vi "Find Channel.vi"(6 "Set":bool, 8 "error in":errorcluster, 10 "Name in":string, 11 "MLTFNC in":refnum<class "MLTFNC.lvclass">) -> (0 "error out":errorcluster, 3 "MLTFNC out":refnum<class "MLTFNC.lvclass">)   [LabVIEW 2019, in "MLTFNC.lvlib" / "MLTFNC.lvclass"]
uses:
  Library/MLTFNC.lvclass
  Library/MLTFNC.lvclass/MLTFNC.ctl
  Accessors/Read Names.vi
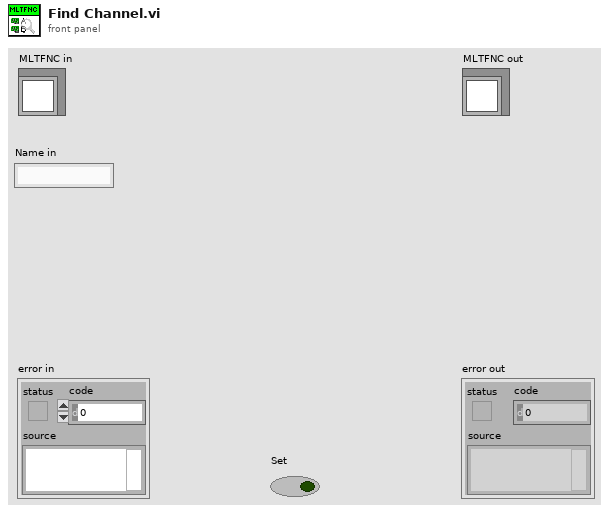
[diagram p1: front panel]
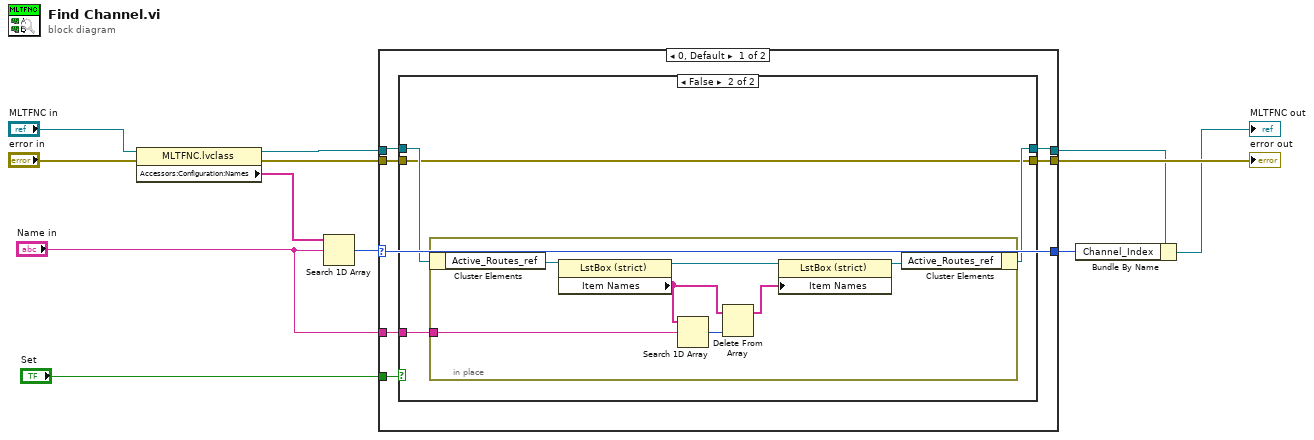
[diagram p0: block diagram]
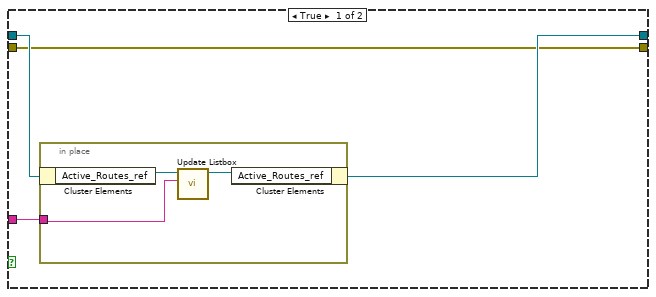
[diagram p2: hidden frame]
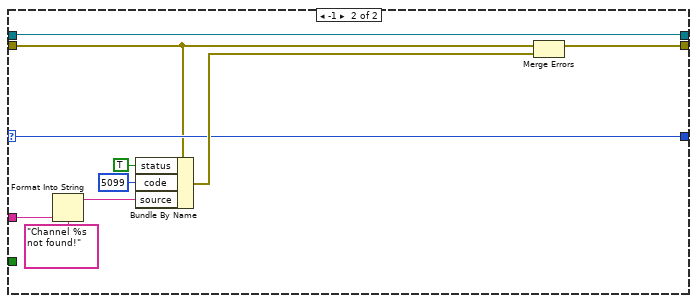
[diagram p3: hidden frame]
diagram:
  n1 = property class="MLTFNC.lvclass"(reference="MLTFNC in", error in="error in") -> (reference out=w5:refnum<class "MLTFNC.lvclass">, error out=w12:errorcluster, "Accessors:Configuration:Names"=w10:string[])
  n2 = Search 1D Array(1D array=w10, element="Name in") -> (index of element=w11:i32)  [unwired: 1 in]
  n3 = case shown="0, Default" w11 {
    selector: w11 -> [w19 w41]
    tunnel: [w19 w41] -> w2
    tunnel: w12 -> [w15 w38]
    tunnel: [w13 w39] -> w6
    tunnel: "Name in" -> [w14 w42]
    tunnel: w5 -> [w18 w40]
    tunnel: [w17 w40] -> w4
    tunnel: "Set" -> [w16 _]
    frame 0, Default {
      n4 = case shown="False" w16 {
        tunnel: w18 -> [w23 w30]
        tunnel: [w22 w29] -> w17
        tunnel: w15 -> [w20 w27]
        tunnel: w14 -> [w21 w28]
        tunnel: [w20 w27] -> w13
        frame True {
          n5 = in-place {
            in-place-border: w21 -> [w24]
            n6 = in-place-cluster #1(w23) -> ("Active_Routes_ref"=w26:refnum<vi>)
            n7 = call "Update Listbox.vi"("Route Target"=w24, "referencein"=w26) -> ("reference out"=w25:refnum<vi>)  [unwired: 9 in]
            n8 = in-place-cluster #1("Active_Routes_ref"=w25) -> (w22:refnum<class "MLTFNC.lvclass">)
          }
        }
        frame False {
          n9 = in-place {
            in-place-border: w28 -> [w34]
            n10 = in-place-cluster #2(w30) -> ("Active_Routes_ref"=w37:refnum<vi>)
            n11 = property class="LstBox (strict)"(reference=w37) -> (reference out=w35:refnum<vi>, "Item Names"=w33:string[])  [unwired: 1 in, 1 out]
            n12 = Search 1D Array(1D array=w33, element=w34) -> (index of element=w32:i32)  [unwired: 1 in]
            n13 = Delete From Array(array=w33, index=w32) -> (array with subset deleted=w31:string[])  [unwired: 1 in, 1 out]
            n14 = property class="LstBox (strict)"(reference=w35, "Item Names"=w31) -> (reference out=w36:refnum<vi>)  [unwired: 1 in, 1 out]
            n15 = in-place-cluster #2("Active_Routes_ref"=w36) -> (w29:refnum<class "MLTFNC.lvclass">)
          }
        }
      }
    }
    frame -1 {
      n16 = Format Into String(format string="Channel %s not found!", w42) -> (resulting string=w43:string)  [unwired: 2 in, 1 out]
      n17 = Bundle By Name(cluster=w38, "status"=TRUE, "code"=5099, "source"=w43) -> (w47:errorcluster)
      n18 = Merge Errors(w38, w47) -> (w39:errorcluster)
    }
  }
  "error out" <- w6
  n19 = Bundle By Name(cluster=w4, "Channel_Index"=w2) -> (→"MLTFNC out":refnum<class "MLTFNC.lvclass">)
